vi "GA_Calculate Fitnesses.vi"(7 "Fitness Function":T2, 11 "Population in":T1) -> (3 "Population out":T1)   [LabVIEW 2016, in "GA.lvlib"]
uses:
  GA.lvlib
  GA_tFitness Function.ctl
  4. Accuracy Assessment for EEG Classification/_vlib/ClassifierClass.lvclass
  GA_tPopulation.ctl
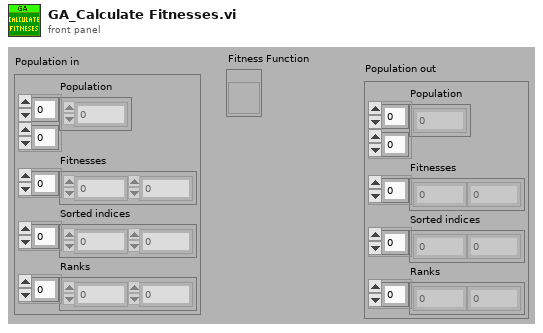
[diagram p1: front panel]
types:
  T1 = typedef "GA.lvlib/GA_tPopulation.ctl" = cluster{"Population":i8[][], "Fitnesses":dbl[], "Sorted indices":i32[], "Ranks":i32[]}
  T2 = typedef "GA.lvlib/GA_tFitness Function.ctl" = refnum<vi>
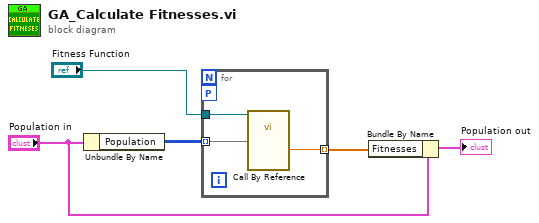
[diagram p0: block diagram]
diagram:
  n1 = Unbundle By Name("Population in") -> ("Population"=w5:i8[][])
  n2 = for {
    tunnel: w5 -> [w7] mode=indexing
    tunnel: "Fitness Function" -> [w8]
    tunnel: [w6] -> w2 mode=indexing
    workers-P: _ -> [_]
    n3 = call-by-ref "?"(reference=w8, "Phenotype"=w7) -> ("Fitness"=w6:dbl)  [unwired: 3 in, 2 out]
  }
  n4 = Bundle By Name(cluster="Population in", "Fitnesses"=w2) -> (→"Population out":T1)
